vi "Toggle2v2.vi"(1 "Initial State":bool, 2 "Reset":bool, 3 "Trigger":bool) -> (0 "New State":bool)   [LabVIEW 2020]
doc: "When the Trigger input is set to TRUE (rising edge), the output New State toggles its Boolean value. The Initial Value of the state can be configured."
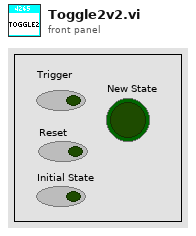
[diagram p1: front panel]
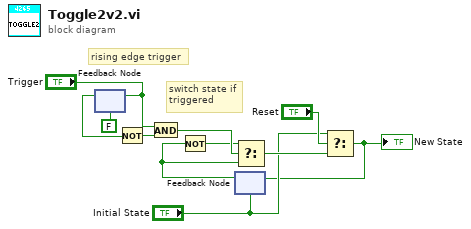
[diagram p0: block diagram]
diagram:
  # "rising edge trigger"
  # "switch state if\ntriggered"
  n1 = feedback-in #1("Trigger") -> ()
  n2 = feedback #1(FALSE ("Button")) -> (w7:bool)
  n3 = Not(x=w7) -> (.not. x?=w9:bool)
  n4 = And(x="Trigger", y=w9) -> (x .and. y?=w11:bool)
  n5 = feedback #2("Initial State") -> (w6:bool)
  n6 = Not(x=w6) -> (.not. x?=w10:bool)
  n7 = Select(t=w10, s=w11, f=w6) -> (s? t:f=w3:bool)
  n8 = Select(t="Initial State", s="Reset", f=w3) -> (s? t:f=w1:bool)
  "New State" <- w1
  n9 = feedback-in #2(w1) -> ()
